vi "ZAlign_Draw_ConnectorPane_DecoFrame.vi"(8 "RightPos":u32[](array[numeric]) caption="Array in", 9 "Bottom":u32, 11 "Panel in":refnum<vi>) -> (0 "Deco refs":refnum<vi>[](array[refnum]), 2 "Decoration out":refnum<vi>, 3 "owner refnumout":refnum<vi>, 5 "rect":T1)   [LabVIEW 2014, in "ZAlign.lvlib"]
doc: "ZAlign.lvlib:ZAlign_Draw_ConnectorPane_DecoFrame.vi\n----------------------------------------------\nDraw ConnectorPane Decoframe\n\nInputs:\n---------------------\n- Array in : 1DArrayOfU32; \n- Bottom : U32; \n- Panel in : Refnum; \n\nOutputs:\n---------------------\n- Deco refs : 1DArrayOfRefnum; \n- rect : Cluster; \n- owner refnumout : Refnum; \n- Decoration out : Refnum; \n\n----------------------------------------------\n16/03/2015\nZühlke Engineering AG\nCH-8952 Schlieren\nwww.zuehlke.com"
uses:
  ZAlign.lvlib
panel:
  # "Connector Pane"
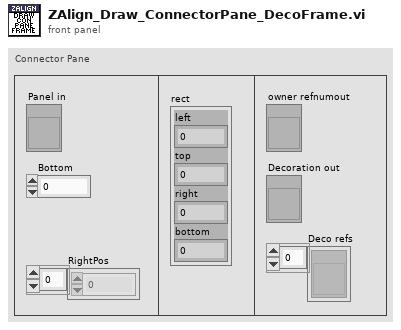
[diagram p1: front panel]
types:
  T1 = cluster{"left":i16, "top":i16, "right":i16, "bottom":i16}
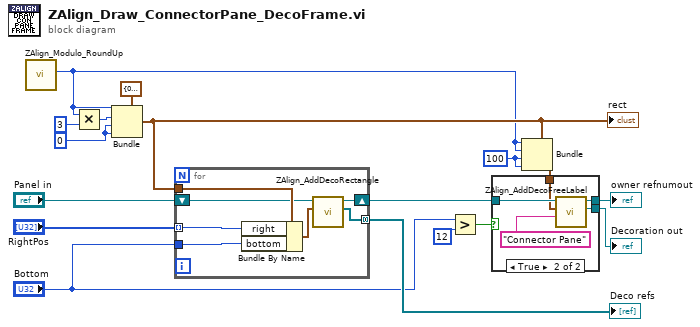
[diagram p0: block diagram]
diagram:
  w5 = i16 100 ("right")
  w10 = i16 0 ("y")
  n1 = call "ZAlign_Modulo_RoundUp.vi"() -> ("Grid_Size"=w6:i32)  [unwired: 10 in, 1 out]
  n2 = Multiply(x=w6, y=i16 3) -> (x*y=w11:i32)
  n3 = Bundle(cluster=T1 {"left"=0, "top"=0, "right"=0, "bottom"=0} ("rect"), "left"=w6, "top"=w11, "right"=w10, "bottom"=w10) -> (w8:T1)
  "rect" <- w8
  n4 = for {
    tunnel: w8 -> [w24]
    tunnel: "Bottom" -> [w23]
    tunnel: "RightPos" -> [w18] mode=indexing
    shift-right: [w22] -> w14
    shift-left: "Panel in" -> [w21]
    tunnel: [w19] -> w4 mode=concatenating
    n5 = Bundle By Name(cluster=w24, "right"=w18, "bottom"=w23) -> (w20:T1)
    n6 = call "ZAlign_AddDecoRectangle.vi"("rect"=w20, "owner refnum"=w21) -> ("Decoration refnums"=w19:refnum<vi>[], "owner refnumout"=w22:refnum<vi>)  [unwired: 7 in, 1 out]
  }
  "Deco refs" <- w4
  n7 = Greater?(x="Bottom", y=12) -> (0:w3:bool)
  n8 = Bundle(cluster=w8, "left"=w6, "top"=w6, "right"=w5, "bottom"=w5) -> (w7:T1)
  n9 = case shown="True" w3 {
    tunnel: [_ w30] -> w16
    tunnel: [w25 w28] -> w15
    tunnel: w14 -> [w25 w27]
    tunnel: w7 -> [_ w26]
    frame False {
    }
    frame True {
      n10 = call "ZAlign_AddDecoFreeLabel.vi"("Text"="Connector Pane", "rect"=w26, "owner refnum"=w27) -> ("Decoration refnum"=w30:refnum<vi>, "owner refnumout"=w28:refnum<vi>)  [unwired: 6 in, 1 out]
    }
  }
  "Decoration out" <- w16
  "owner refnumout" <- w15
